vi "Sub Super Duper_14_02_12_JWa.vi"(0 "VISA resource name":refnum<visa-resource-name>="GPIB0::17::INSTR", 1 "Sample Properties:":T9 {"Date Created" format="%<%Y/%m/%d>T"}, 2 "Gated SMU4 is...":bool, 3 "TRF Cluster":T10={"Step 4"=-38.0, "# of Loops"=1.0, "Transfer 2"=FALSE, "Start 4"=-2.0, "Total Points 2"=2, "Start 3"=40.0, "Stop 2"=-40.0, "Step 3"=-1.0, "Loop Step"=0.0, "Integration Time 3"=0, "Loop Wait"=0.0, "First Step"=0.0} {"Loop Wait" format="%<%H:%M:%S>t"; "Integration Time 3" scale=0.0..2.0; "Step 3" format="%.2f"; "Stop 2" format="%.2f"; "Start 3" format="%.2f"; "Start 4" format="%.2f"; "Step 4" format="%.2f"}, 4 "TSP Cluster":T11={"Transport"=FALSE, "Start 2"=0.0, "Stop 3"=-60.0, "Step 2"=-1.0, "Start"=0.0, "Step"=-10.0, "Total Points"=7, "Integration Time"=0} {"Integration Time" scale=0.0..2.0; "Step" format="%.2f"; "Start" format="%.2f"; "Step 2" format="%.2f"; "Stop 3" format="%.2f"; "Start 2" format="%.2f"}, 5 "Compliance Cluster":T6={"Var1 sweep settings"={"sweep spacing (linear: 0)"=0, "sweep mode"=FALSE, "compliance (V)"=100.0, "compliance (A)"=0.001}, "Var1 sweep settings 2"={"sweep spacing (linear: 0)"=0, "sweep mode"=FALSE, "compliance (V)"=100.0, "compliance (A)"=0.001}, "Var2 step settings 2"={"compliance (A)"=0.001, "compliance (V)"=100.0}, "Var2 step settings"={"compliance (A)"=0.001, "compliance (V)"=100.0}} {"Var2 step settings"."compliance (V)" format="%.2f"; "Var2 step settings"."compliance (A)" format="%^.2e"; "Var2 step settings 2"."compliance (V)" format="%.2f"; "Var2 step settings 2"."compliance (A)" format="%^.2e"; "Var1 sweep settings 2"."compliance (A)" format="%^.2e"; "Var1 sweep settings 2"."compliance (V)" format="%.2f"; "Var1 sweep settings 2"."sweep spacing (linear: 0)" items=["linear", "log 10", "log 25", "log 50"]; "Var1 sweep settings"."compliance (A)" format="%^.2e"; "Var1 sweep settings"."compliance (V)" format="%.2f"; "Var1 sweep settings"."sweep spacing (linear: 0)" items=["linear", "log 10", "log 25", "log 50"]}, 6 "Light Bathe Cluster":T2={"TG to BG:  "=FALSE, "TG to BG Durration"=120.0, "TRF to TSP:   "=FALSE, "TRF to TSP Duration"=120.0, "Post Measure: "=FALSE, "TG to BG (TSP):"=FALSE, "TG to BG Durration 3"=120.0} {"TG to BG Durration 3" format="%<%H:%M:%S>t"; "TRF to TSP Duration" format="%<%H:%M:%S>t"; "TG to BG Durration" format="%<%H:%M:%S>t"}, 7 "error in":errorcluster, 8 "Saved Folder:":path=path "C:/1DATA/2011", 9 "Wait Cluster":T5 {"Wait Time (s)" format="%.1g"; "Wait Countdown" format="%<%H:%M:%S%1u>t"}, 13 "Stop \nCountdown":bool, 15 "Loop Count":dbl, 16 "Gate Current Cluster":T3={"Gate Current (TSP)"={"Y2 axis on/off"=FALSE, "MINIMUM"=0.0, "MAXIMUM"=1.0, "Variable name"="Ig", "LIN or LOG axis"="LIN"}, "Gate Current (TRF)"={"Y2 axis on/off"=FALSE, "MINIMUM"=0.0, "MAXIMUM"=1.0, "Variable name"="Ig", "LIN or LOG axis"="LIN"}} {"Gate Current (TSP)"."MAXIMUM" format="%.9f"; "Gate Current (TSP)"."MINIMUM" format="%.9f"; "Gate Current (TRF)"."MAXIMUM" format="%.9f"; "Gate Current (TRF)"."MINIMUM" format="%.9f"}, 17 "Dielectric Constant (BG)":dbl) -> (12 "Status Indicator":bool, 14 "Vt Cluster":T4 {"Id Max" format="%.3g"; "Vt Max" format="%.3g"; "Vt Min" format="%.3g"; "Vt Ratio" format="%.3g"}, 20 "VISA resource name out":refnum<visa-resource-name>, 21 "TRF Path":path, 23 "TSP Path":path, 24 "Graph Cluster":T7, 25 "Char Cluster":T8 {"Mobility-Lin" format="%#_4e"; "On/Off" format="%#_4e"; "Mobility-Sat" format="%#_4e"}, 27 "error out":errorcluster)   [LabVIEW 2012]
uses:
  <vilib>/Platform/TimedLoop/XDataNode/wakeup.ctl
  <vilib>/Platform/TimedLoop/XDataNode/XDNodeRunTimeDep.lvlib
  <vilib>/Platform/TimedLoop/XDataNode/nitl_modes.ctl
  <vilib>/Platform/TimedLoop/XDataNode/timing_clust.ctl
  <vilib>/Platform/TimedLoop/XDataNode/XDataNode.xnode
panel:
  in  "TG Dielectric Prop":T1
  out "LKG Path":path
  # "Vg Sweep"
  # "Vd Step"
  # "Loops and Integration Time"
  # "Device Characteristics"
  # "Light Bath is..."
  # "Duration (hh:mm:ss)"
  # "Sample Properties:"
  # "%"
  # "nm"
  # "Device Properties:"
  # "um"
  # "um"
  # "Vg Step"
  # "Vd Step"
  # "Integration Time"
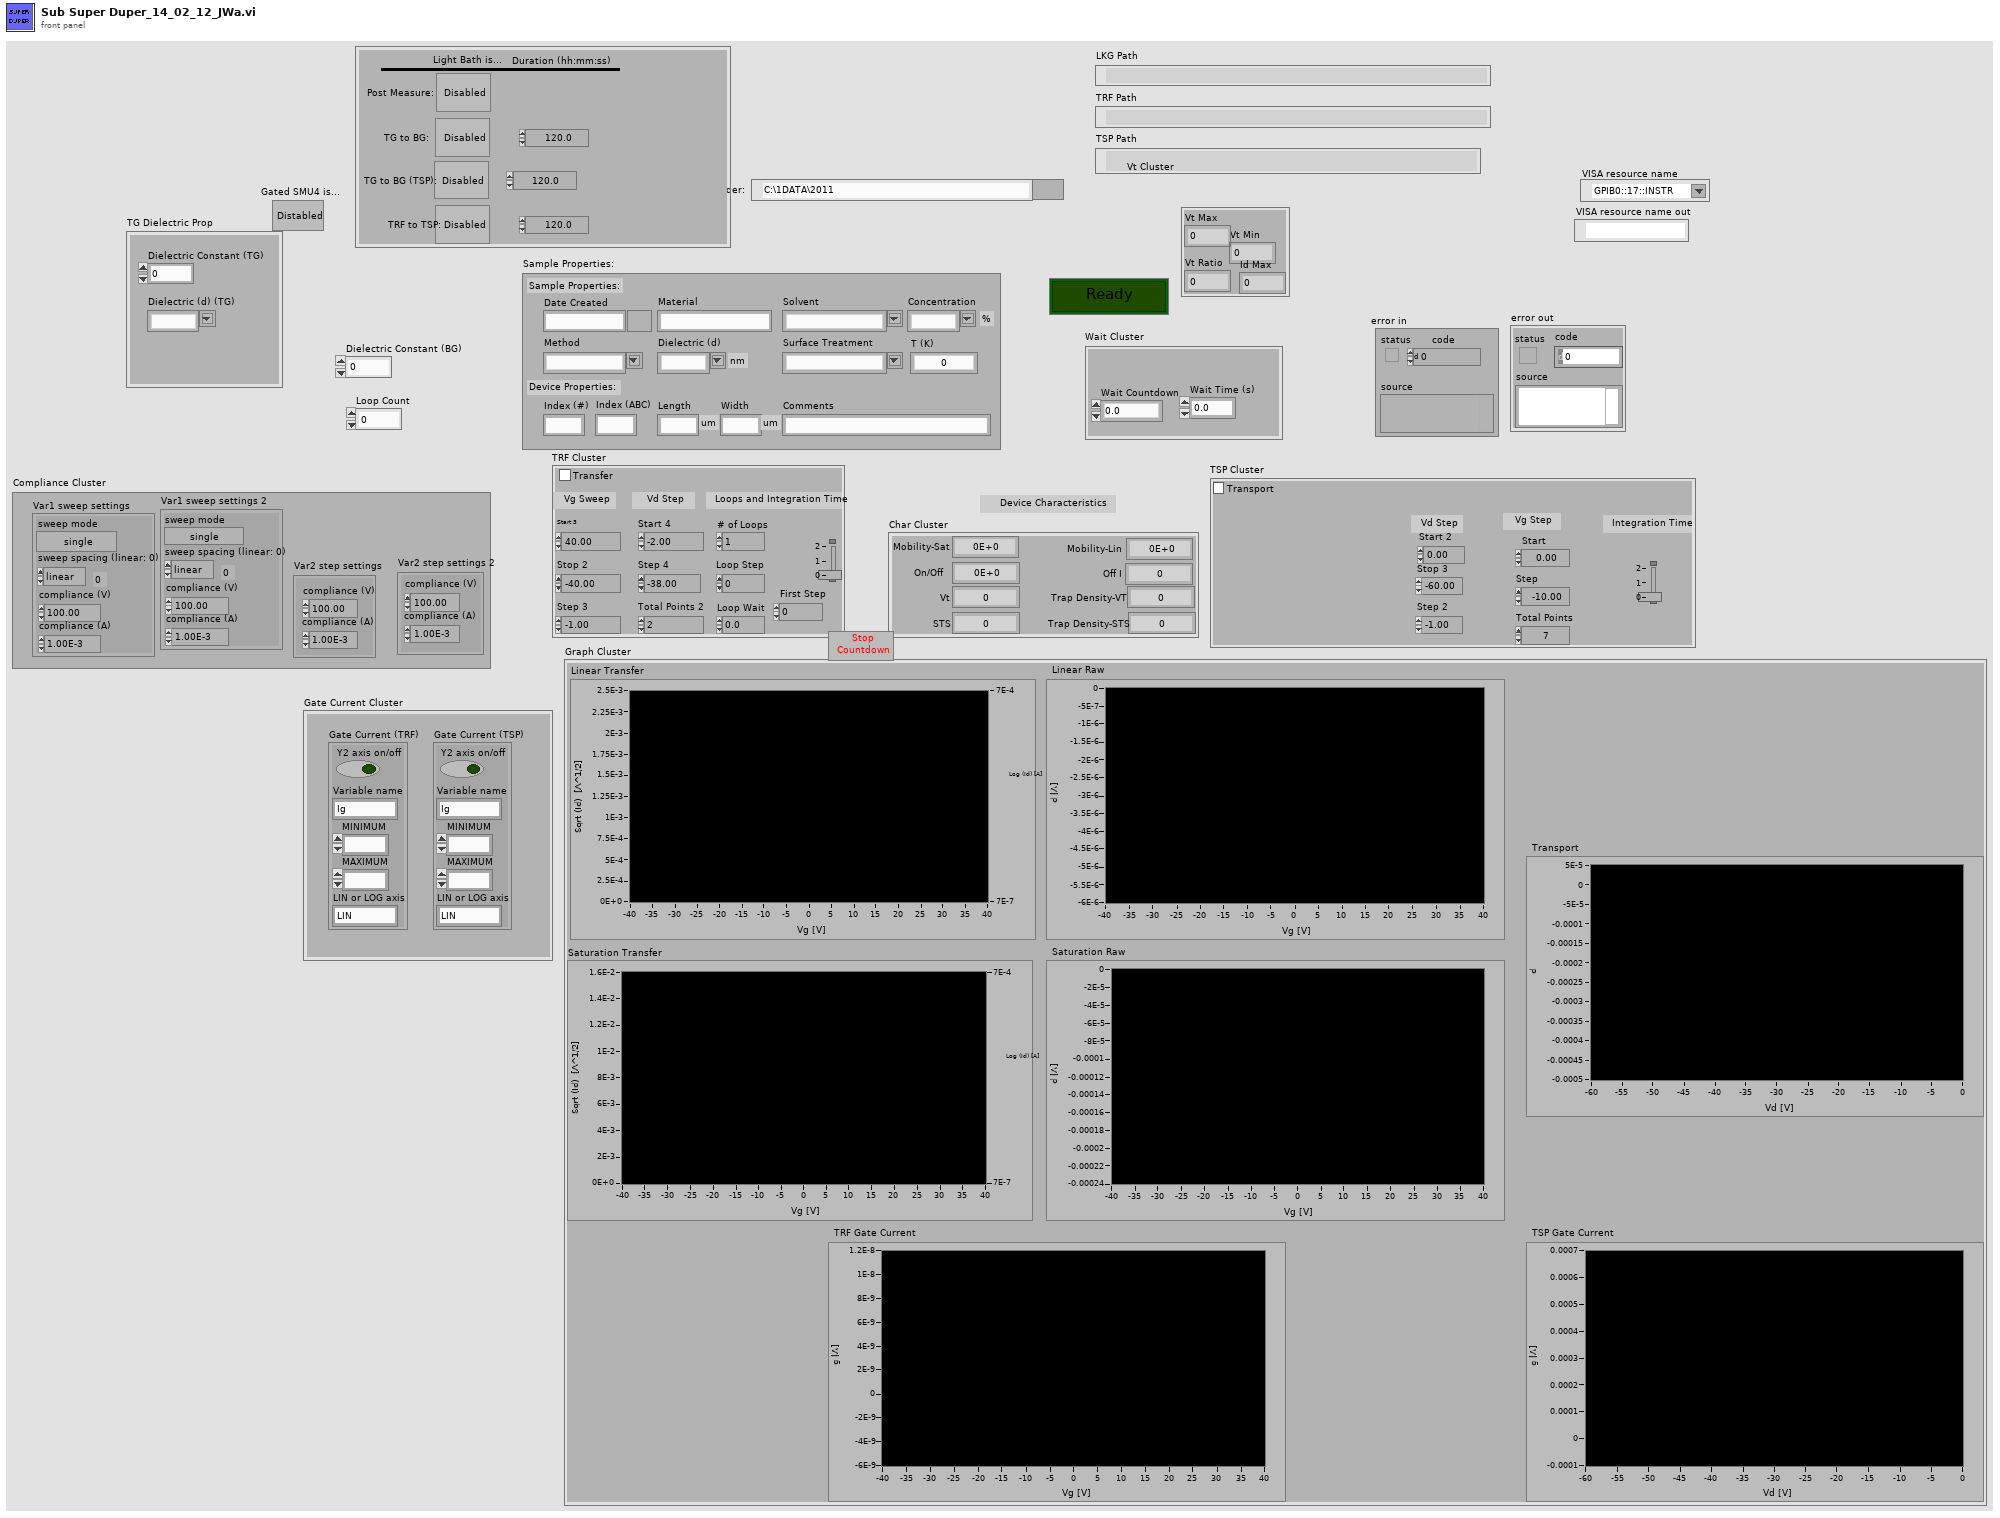
[diagram p1: front panel]
types:
  T1 = cluster{"Dielectric Constant (TG)":dbl, "Dielectric (d) (TG)":string}
  T2 = cluster{"TG to BG:  ":bool, "TG to BG Durration":dbl, "TRF to TSP:   ":bool, "TRF to TSP Duration":dbl, "Post Measure: ":bool, "TG to BG (TSP):":bool, "TG to BG Durration 3":dbl}
  T3 = cluster{"Gate Current (TSP)":cluster{"Y2 axis on/off":bool, "MINIMUM":ext, "MAXIMUM":ext, "Variable name":string, "LIN or LOG axis":string}, "Gate Current (TRF)":cluster{"Y2 axis on/off":bool, "MINIMUM":ext, "MAXIMUM":ext, "Variable name":string, "LIN or LOG axis":string}}
  T4 = cluster{"Vt Max":i32, "Vt Min":i32, "Vt Ratio":i32, "Id Max":i32}
  T5 = cluster{"Wait Countdown":dbl, "Wait Time (s)":dbl}
  T6 = cluster{"Var1 sweep settings":cluster{"sweep spacing (linear: 0)":u16, "sweep mode":bool, "compliance (V)":dbl, "compliance (A)":dbl}, "Var1 sweep settings 2":cluster{"sweep spacing (linear: 0)":u16, "sweep mode":bool, "compliance (V)":dbl, "compliance (A)":dbl}, "Var2 step settings 2":cluster{"compliance (A)":dbl, "compliance (V)":dbl}, "Var2 step settings":cluster{"compliance (A)":dbl, "compliance (V)":dbl}}
  T7 = cluster{"Linear Transfer":cluster{dbl[], "trace":dbl[]}[], "Linear Raw":cluster{dbl[], dbl[]}[], "Saturation Transfer":cluster{dbl[], "trace":dbl[]}[], "Saturation Raw":cluster{dbl[], dbl[]}[], "Transport":cluster{dbl[], dbl[]}[], "TRF Gate Current":cluster{dbl[], dbl[]}[], "TSP Gate Current":cluster{dbl[], dbl[]}[]}
  T8 = cluster{"Mobility-Sat":dbl, "Mobility-Lin":dbl, "On/Off ":dbl, "Off I":dbl, "Vt":dbl, "STS":dbl, "Trap Density-VT":dbl, "Trap Density-STS":dbl}
  T9 = cluster{"Date Created":timestamp, "Material":string, "Solvent":string, "Concentration":string, "Method":string, "Dielectric (d)":string, "Index (#)":string, "Index (ABC)":string, "Length":string, "Width":string, "Surface Treatment":string, "Comments":string, "T (K)":dbl}
  T10 = cluster{"Step 4":dbl, "# of Loops":dbl, "Transfer 2":bool, "Start 4":dbl, "Total Points 2":u16, "Start 3":dbl, "Stop 2":dbl, "Step 3":dbl, "Loop Step":dbl, "Integration Time 3":u32, "Loop Wait":dbl, "First Step":dbl}
  T11 = cluster{"Transport":bool, "Start 2":dbl, "Stop 3":dbl, "Step 2":dbl, "Start":dbl, "Step":dbl, "Total Points":u16, "Integration Time":u32}
  T12 = typedef "XDNodeRunTimeDep.lvlib/timing_clust.ctl" = cluster{"Expected End [f-1]":u64, "Actual End [f-1]":u64, "Finished Late? [f-1]":bool, "Expected End [i-1]":u64, "Actual End [i-1]":u64, "Finished Late? [i-1]":bool, "Expected Start [i]":u64, "Actual Start [i]":u64, "Expected Start [f]":u64, "Actual Start [f]":u64, "Source Name":string, "Structure Name":string, "Period":i64, "Deadline":i64, "Offset":i64, "Start":i64, "Priority":i32, "Timeout":i32, "Mode":T13, "Wakeup Reason":T14, "Error":errorcluster, "Source Type":string, "Secondary Source Type":string, "Global End Time":u64, "Global Start Time":u64, "Frame Duration":u64, "Iteration Duration":u64, "Assigned CPU":i32, "I/O Scan Engine Mode":u32}
  T13 = typedef "XDNodeRunTimeDep.lvlib/nitl_modes.ctl" = enum32{"No Change", "Process missed periods, maintain original phase", "Discard missed periods, maintain original phase", "Process missed periods, ignore original phase", "Discard missed periods, ignore original phase"}
  T14 = typedef "XDNodeRunTimeDep.lvlib/wakeup.ctl" = enum32{"Normal", "Aborted", "Asynchronous wakeup", "Timing source error", "Timed loop error", "Timeout"}
  T15 = cluster{"sweep spacing (linear: 0)":u16, "sweep mode":bool, "compliance (V)":dbl, "compliance (A)":dbl}
  T16 = cluster{"compliance (A)":dbl, "compliance (V)":dbl}
  T17 = cluster{"Y2 axis on/off":bool, "MINIMUM":ext, "MAXIMUM":ext, "Variable name":string, "LIN or LOG axis":string}
  T18 = cluster{"Start 3":dbl, "Stop 2":dbl, "Step 3":dbl, "sweep spacing (linear: 0)":u16, "sweep mode":bool, "compliance (V)":dbl, "compliance (A)":dbl}
  T19 = cluster{"compliance (A)":dbl, "compliance (V)":dbl, "Start 4":dbl, "Total Points 2":u16, dbl}
  T20 = cluster{"Vt Max":i32, "Vt Min":i32, "Vt Ratio":i32, "Id Max":dbl}
  T21 = cluster{"Mobility-Sat":dbl, "Mobility-Lin":dbl, "On/Off Current":dbl, "Off I":dbl, "Vt":dbl, "STS":dbl, "Trap Density-VT":dbl, "Trap Density-STS":dbl}
  T22 = cluster{"Linear Sqrt":cluster{dbl[], "trace":dbl[]}[], "Linear Log":cluster{dbl[], "trace":dbl[]}[], "Linear Raw":cluster{dbl[], dbl[]}[], "Saturation Sqrt":cluster{dbl[], "trace":dbl[]}[], "Saturation Log":cluster{dbl[], "trace":dbl[]}[], "Saturation Raw":cluster{dbl[], "trace":dbl[]}[], "Gate Current":cluster{dbl[], "trace":dbl[]}[]}
  T23 = cluster{"Start 2":dbl, "Stop 3":dbl, "Step 2":dbl, "sweep spacing (linear: 0)":u16, "sweep mode":bool, "compliance (V)":dbl, "compliance (A)":dbl}
  T24 = cluster{"compliance (A)":dbl, "compliance (V)":dbl, "Start":dbl, "Total Points":u16, "Step":dbl}
  T25 = cluster{"Transport":cluster{dbl[], dbl[]}[], "Gate Current":cluster{dbl[], dbl[]}[]}
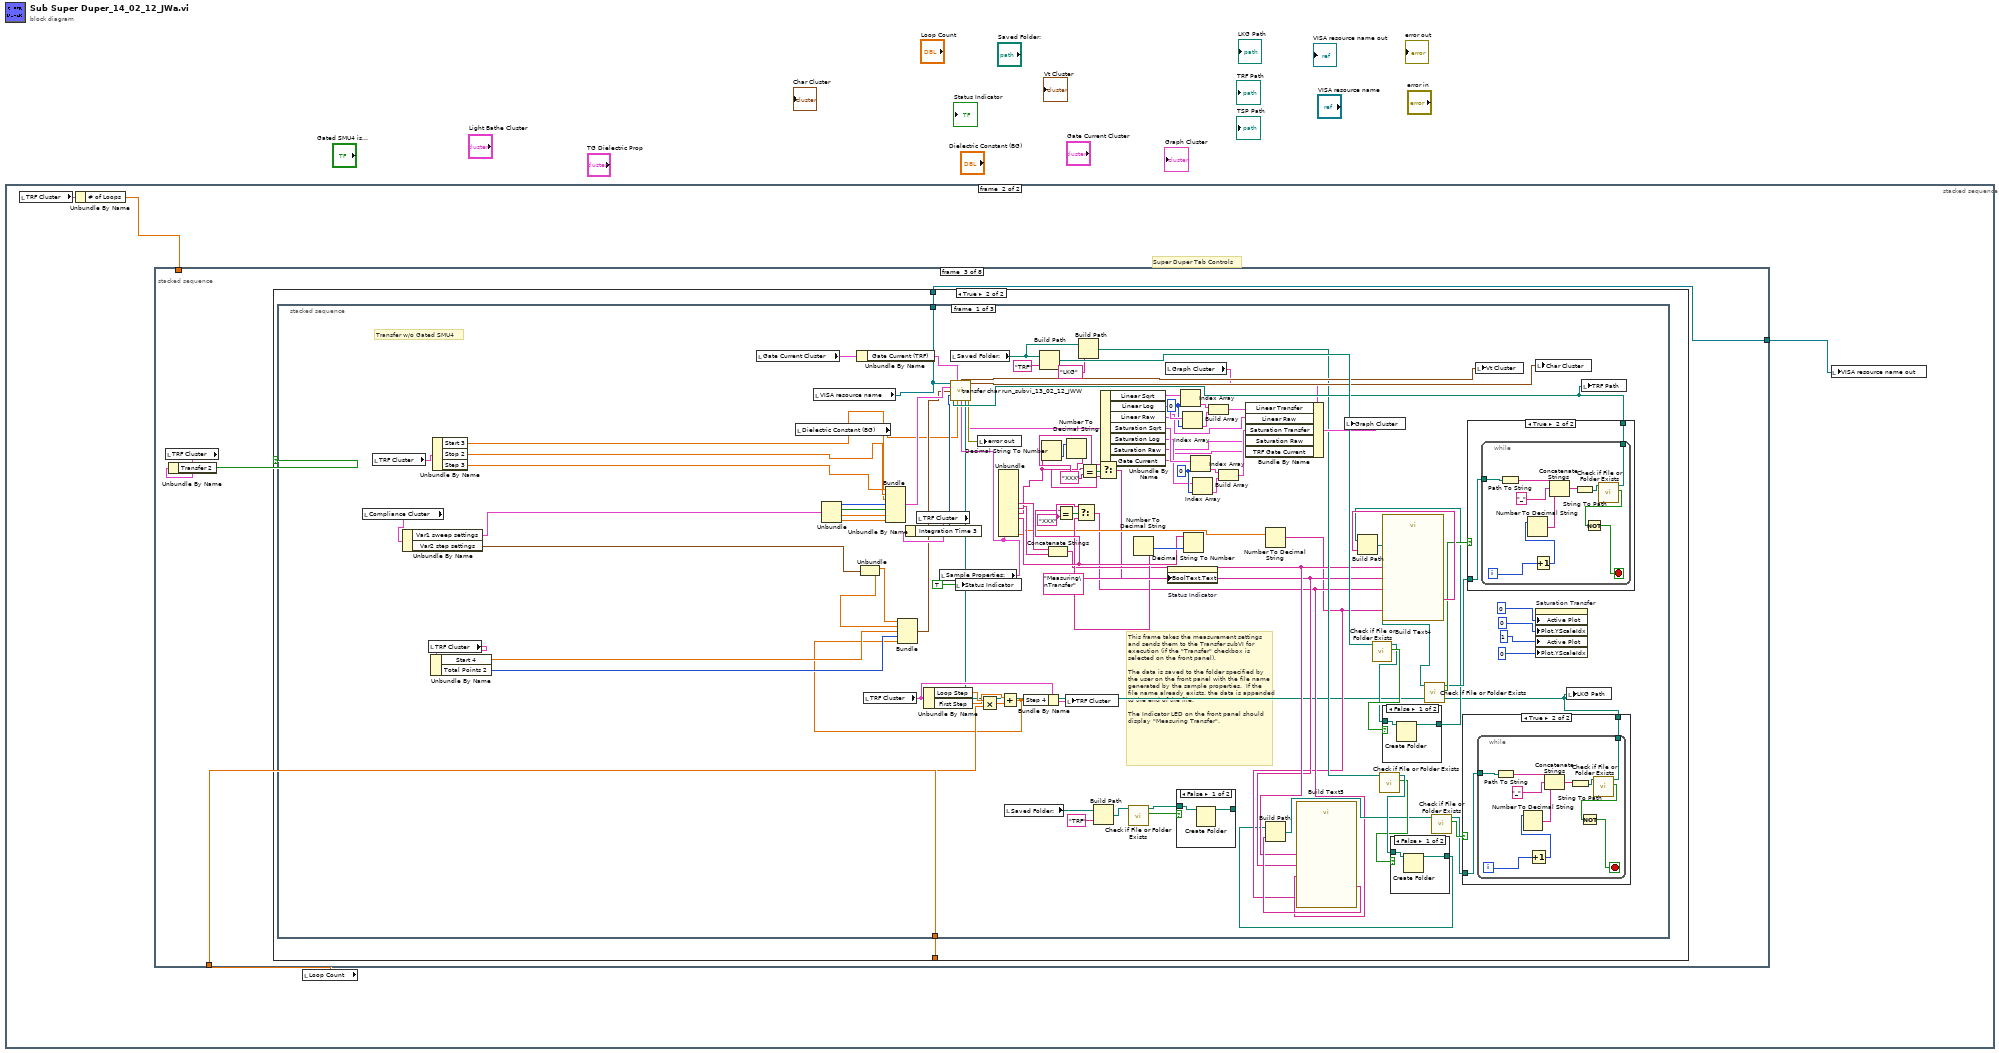
[diagram p0: block diagram]
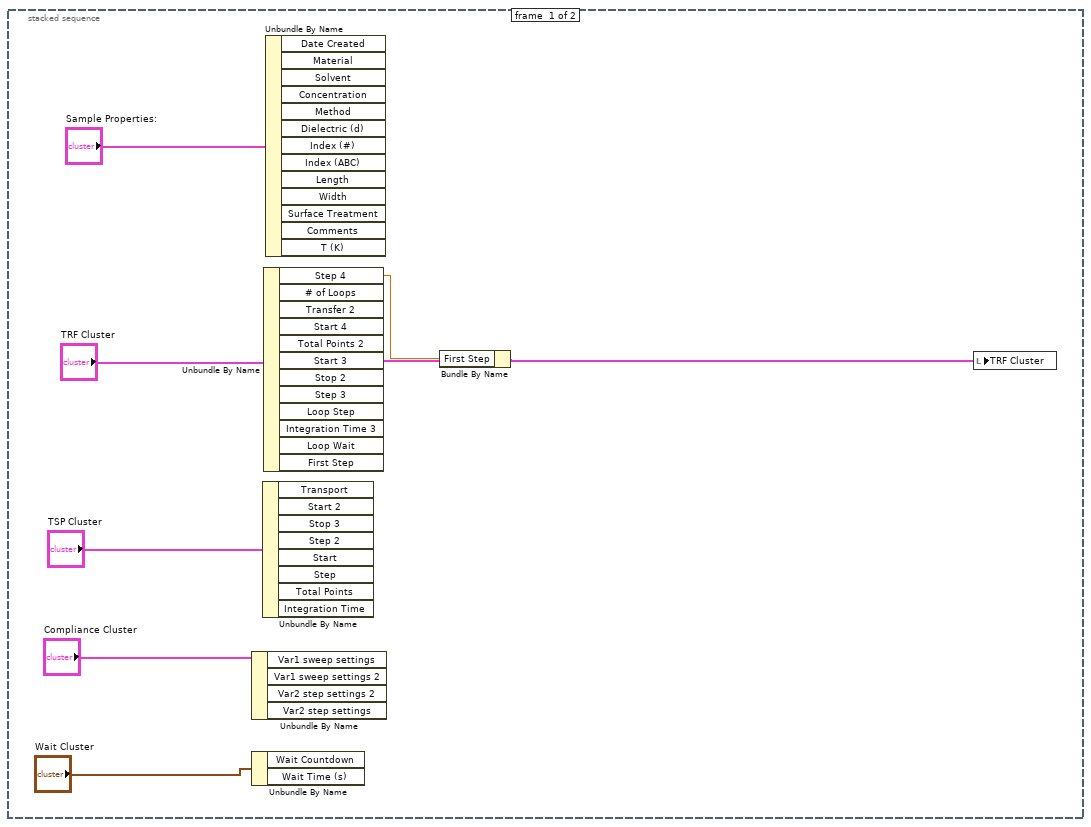
[diagram p2: hidden frame]
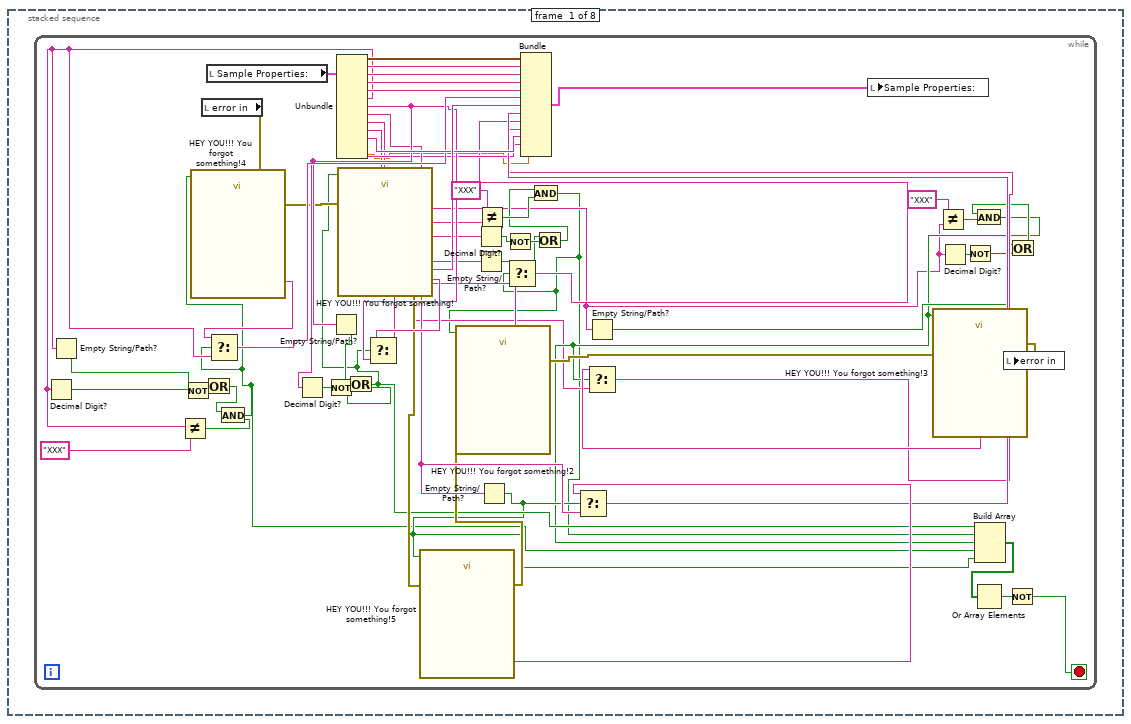
[diagram p3: hidden frame]
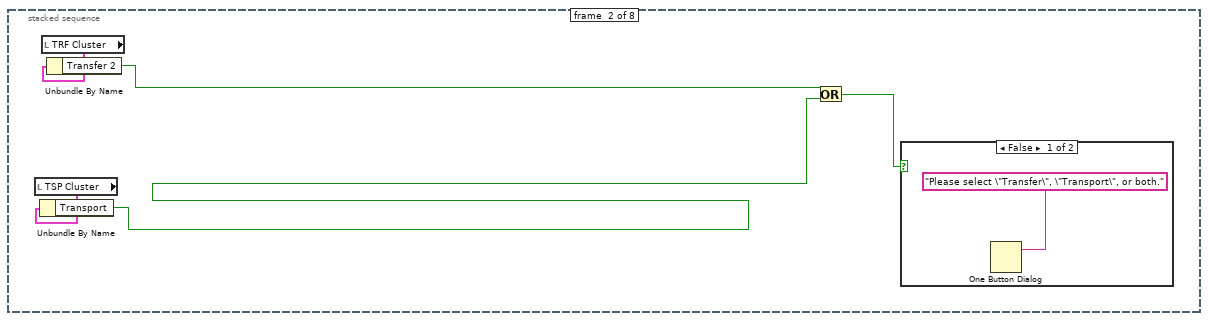
[diagram p4: hidden frame]
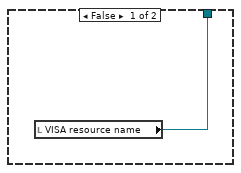
[diagram p6: hidden frame]
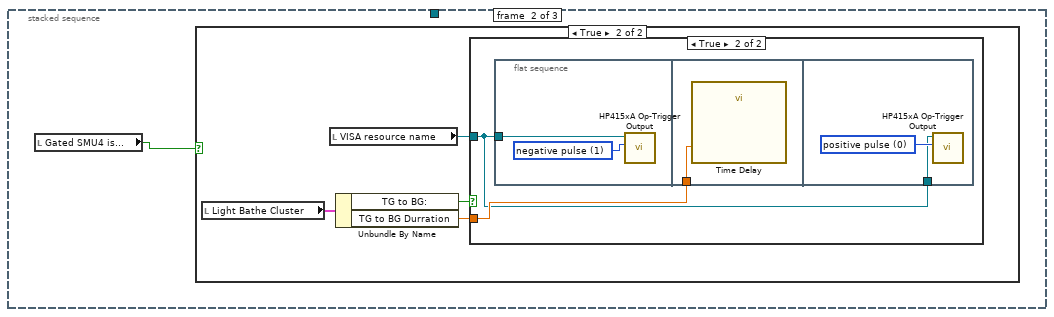
[diagram p12: hidden frame]
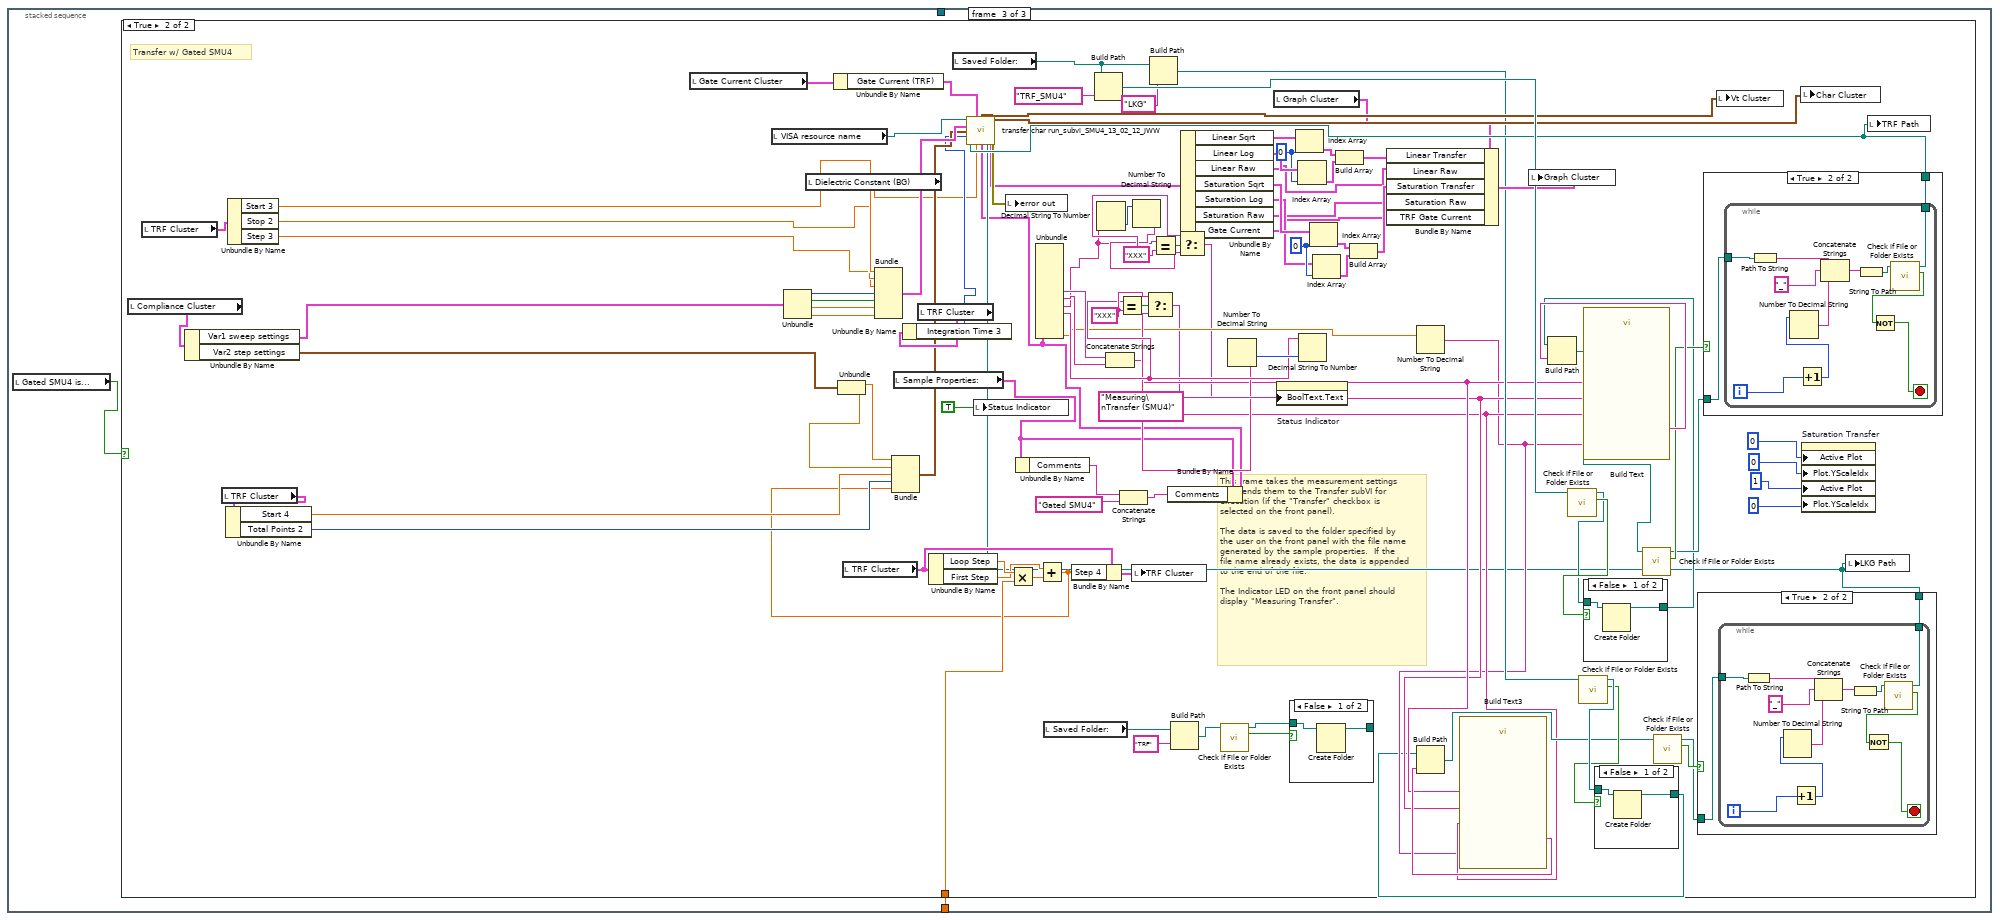
[diagram p15: hidden frame]
diagram:
  n1 = stacked-sequence {
    frame #0 {
      n2 = Unbundle By Name("Compliance Cluster") -> ()  [unwired: 4 out]
      n3 = Unbundle By Name("Wait Cluster") -> ()  [unwired: 2 out]
      n4 = Unbundle By Name("TSP Cluster") -> ()  [unwired: 8 out]
      n5 = Unbundle By Name("TRF Cluster") -> ("Step 4"=w7:dbl)  [unwired: 11 out]
      n6 = Unbundle By Name("Sample Properties:") -> ()  [unwired: 13 out]
      n7 = Bundle By Name(cluster="TRF Cluster", "First Step"=w7) -> (w5:T10)
      n8 = local write "TRF Cluster"(w5) -> ()
    }
    frame #1 {
      # "Super Duper Tab Controls"
      n9 = local read "TRF Cluster"() -> (w11:T10)
      n10 = Unbundle By Name(w11) -> ("# of Loops"=w10:dbl)
      n11 = local read "Loop Count"() -> (w8:dbl)
      n12 = stacked-sequence {
        tunnel: w8 -> [_ _ w81 _ _ _ _ w593]
        tunnel: w10 -> [_ _ _ _ _ _ _ w592]
        tunnel: [_ _ w78 _ _ _ _ _] -> w9
        frame #0 {
          n13 = while {
            stop <- w37 stop-if-true
            n14 = local read "error in"() -> (w43:errorcluster)
            n15 = local read "Sample Properties:"() -> (w66:T9)
            n16 = Unbundle(w66) -> ("Date Created"=w67:timestamp, "Material"=w68:string, "Solvent"=w69:string, "Concentration"=w70:string, "Method"=w71:string, "Dielectric (d)"=w26:string, "Index (#)"=w56:string, "Index (ABC)"=w53:string, "Length"=w21:string, "Width"=w14:string, "Surface Treatment"=w59:string, "Comments"=w51:string, "T (K)"=w12:dbl)
            n17 = Decimal Digit?(1:w26) -> (0:w34:bool)
            n18 = Empty String/Path?(string/path=w26) -> (empty?=w28:bool)
            n19 = Not Equal?(x=w26, y="XXX") -> (x != y?=w25:bool)
            n20 = Not(x=w34) -> (.not. x?=w31:bool)
            n21 = Or(x=w28, y=w31) -> (x .or. y?=w24:bool)
            n22 = And(x=w24, y=w25) -> (x .and. y?=w23:bool)
            n23 = call "HEY YOU!!! You forgot something!4"("Enable"=w23, "error in (no error)"=w43) -> ("Dielectric (d)"=w58:string, "error out"=w42:errorcluster)  [unwired: 15 in, 1 out]
            n24 = Select(t=w58, s=w23, f=w26) -> (s? t:f=w57:string)
            n25 = Decimal Digit?(1:w56) -> (0:w47:bool)
            n26 = Not(x=w47) -> (.not. x?=w46:bool)
            n27 = Empty String/Path?(string/path=w56) -> (empty?=w55:bool)
            n28 = Or(x=w55, y=w46) -> (x .or. y?=w41:bool)
            n29 = call "HEY YOU!!! You forgot something!"("Enable"=w41, "error in (no error)"=w42) -> ("Index (#)"=w65:string, "error out"=w45:errorcluster)  [unwired: 15 in, 1 out]
            n30 = Select(t=w65, s=w41, f=w56) -> (s? t:f=w62:string)
            n31 = Decimal Digit?(1:w21) -> (0:w36:bool)
            n32 = Empty String/Path?(string/path=w21) -> (empty?=w30:bool)
            n33 = Not Equal?(x="XXX", y=w21) -> (x != y?=w20:bool)
            n34 = Empty String/Path?(string/path=w53) -> (empty?=w40:bool)
            n35 = call "HEY YOU!!! You forgot something!5"("Enable"=w40, "error in (no error)"=w45) -> ("Index (ABC)"=w54:string, "error out"=w44:errorcluster)  [unwired: 15 in, 1 out]
            n36 = Not(x=w36) -> (.not. x?=w33:bool)
            n37 = Or(x=w30, y=w33) -> (x .or. y?=w19:bool)
            n38 = And(x=w19, y=w20) -> (x .and. y?=w13:bool)
            n39 = call "HEY YOU!!! You forgot something!2"("Enable"=w13, "error in (no error)"=w44) -> ("Length"=w64:string, "error out"=w61:errorcluster)  [unwired: 15 in, 1 out]
            n40 = Select(t=w64, s=w13, f=w21) -> (s? t:f=w50:string)
            n41 = Select(t=w54, s=w40, f=w53) -> (s? t:f=w52:string)
            n42 = Empty String/Path?(string/path=w14) -> (empty?=w29:bool)
            n43 = Not Equal?(x="XXX", y=w14) -> (x != y?=w18:bool)
            n44 = Decimal Digit?(1:w14) -> (0:w35:bool)
            n45 = Not(x=w35) -> (.not. x?=w32:bool)
            n46 = Or(x=w29, y=w32) -> (x .or. y?=w17:bool)
            n47 = And(x=w17, y=w18) -> (x .and. y?=w16:bool)
            n48 = call "HEY YOU!!! You forgot something!3"("Enable"=w16, "error in (no error)"=w61) -> ("Width"=w63:string, "error out"=w60:errorcluster)  [unwired: 15 in, 1 out]
            n49 = Select(t=w63, s=w16, f=w14) -> (s? t:f=w49:string)
            n50 = Bundle("Date Created"=w67, "Material"=w68, "Solvent"=w69, "Concentration"=w70, "Method"=w71, "Dielectric (d)"=w57, "Index (#)"=w62, "Index (ABC)"=w52, "Length"=w50, "Width"=w49, "Surface Treatment"=w59, "Comments"=w51, "T (K)"=w12) -> (w48:T9)  [unwired: 1 in]
            n51 = local write "Sample Properties:"(w48) -> ()
            n52 = Build Array(w41, w13, w16, w23, w40) -> (w39:bool[])
            n53 = Or Array Elements(Boolean array=w39) -> (logical OR=w38:bool)
            n54 = local write "error in"(w60) -> ()
            n55 = Not(x=w38) -> (.not. x?=w37:bool)
          }
        }
        frame #1 {
          n56 = local read "TSP Cluster"() -> (w73:T11)
          n57 = Unbundle By Name(w73) -> ("Transport"=w72:bool)
          n58 = local read "TRF Cluster"() -> (w75:T10)
          n59 = Unbundle By Name(w75) -> ("Transfer 2"=w74:bool)
          n60 = Or(x=w74, y=w72) -> (x .or. y?=w76:bool)
          n61 = case shown="False" w76 {
            frame False {
              n62 = One Button Dialog(message="Please select \"Transfer\", \"Transport\", or both.") -> ()  [unwired: 1 in, 1 out]
            }
            frame True {
            }
          }
        }
        frame #2 {
          n63 = local read "TRF Cluster"() -> (w79:T10)
          n64 = Unbundle By Name(w79) -> ("Transfer 2"=w80:bool)
          n65 = case shown="True" w80 {
            tunnel: w81 -> [_ w84]
            tunnel: [w82 w83] -> w78
            frame False {
              n66 = local read "VISA resource name"() -> (w82:refnum<visa-resource-name>)
            }
            frame True {
              n67 = stacked-sequence {
                tunnel: w84 -> [w186 _ w237]
                tunnel: [w185 _ _] -> w83
                frame #0 {
                  w115 = 0
                  w121 = 0
                  w164 = "XXX"
                  w167 = "XXX"
                  # "Transfer w/o Gated SMU4"
                  # "This frame takes the measurement settings and sends them to the Transfer subVI for execution (if the \"Transfer\" checkbox is selected on the front panel).\n\nThe data is saved to the folder specified by the user on the front panel with the file name generated by the sample properties.  If the file name already exists, the data is appended to the end of the file.\n\nThe Indicator LED on the front panel should display \"Measuring Transfer\"."
                  n68 = local read "Compliance Cluster"() -> (w143:T6)
                  n69 = local read "TRF Cluster"() -> (w148:T10)
                  n70 = Unbundle By Name(w143) -> ("Var1 sweep settings"=w141:T15, "Var2 step settings"=w142:T16)
                  n71 = local read "TRF Cluster"() -> (w151:T10)
                  n72 = Unbundle By Name(w151) -> ("Start 4"=w150:dbl, "Total Points 2"=w149:u16)
                  n73 = Unbundle By Name(w148) -> ("Start 3"=w147:dbl, "Stop 2"=w146:dbl, "Step 3"=w145:dbl)
                  n74 = local read "Gate Current Cluster"() -> (w87:T3)
                  n75 = local read "Dielectric Constant (BG)"() -> (w85:dbl)
                  n76 = local read "VISA resource name"() -> (w185:refnum<visa-resource-name>)
                  n77 = Unbundle(w141) -> ("sweep spacing (linear: 0)"=w184:u16, "sweep mode"=w183:bool, "compliance (V)"=w182:dbl, "compliance (A)"=w181:dbl)
                  n78 = Unbundle By Name(w87) -> ("Gate Current (TRF)"=w86:T17)
                  n79 = Unbundle(w142) -> ("compliance (A)"=w180:dbl, "compliance (V)"=w179:dbl)
                  n80 = local read "TRF Cluster"() -> (w134:T10)
                  n81 = Bundle("Start 3"=w147, "Stop 2"=w146, "Step 3"=w145, "sweep spacing (linear: 0)"=w184, "sweep mode"=w183, "compliance (V)"=w182, "compliance (A)"=w181) -> (w133:T18)  [unwired: 1 in]
                  n82 = local read "TRF Cluster"() -> (w144:T10)
                  n83 = Unbundle By Name(w144) -> ("Integration Time 3"=w131:u32)
                  n84 = Unbundle By Name(w134) -> ("Loop Step"=w137:dbl, "First Step"=w136:dbl)
                  n85 = local read "Sample Properties:"() -> (w129:T9)
                  n86 = local read "Saved Folder:"() -> (w102:path)
                  n87 = local write "Status Indicator"(TRUE) -> ()
                  n88 = Multiply(x=w137, y=w186) -> (x*y=w139:dbl)
                  n89 = Unbundle(w129) -> ("Index (#)"=w175:string, "Index (ABC)"=w174:string, "Length"=w161:string, "Width"=w163:string, "T (K)"=w140:dbl)  [unwired: 8 out]
                  n90 = Add(x=w136, y=w139) -> (x+y=w135:dbl)
                  n91 = Bundle("compliance (A)"=w180, "compliance (V)"=w179, "Start 4"=w150, "Total Points 2"=w149, w135) -> (w132:T19)  [unwired: 1 in]
                  n92 = local read "Saved Folder:"() -> (w108:path)
                  n93 = Bundle By Name(cluster=w134, "Step 4"=w135) -> (w138:T10)
                  n94 = Build Path(base path=w102, name or relative path="TRF") -> (appended path=w157:path)
                  n95 = Decimal String To Number(string=w161) -> (number=w170:i32)  [unwired: 2 in, 1 out]
                  n96 = Concatenate Strings(w175, w174) -> (w93:string)
                  n97 = Equal?(x=w163, y=w164) -> (x = y?=w165:bool)
                  n98 = local write "TRF Cluster"(w138) -> ()
                  n99 = Number To Decimal String(number=w170) -> (decimal integer string=w166:string)  [unwired: 1 in]
                  n100 = Build Path(base path=w102, name or relative path="LKG") -> (appended path=w98:path)
                  n101 = Equal?(x=w161, y=w167) -> (x = y?=w168:bool)
                  n102 = Build Path(base path=w108, name or relative path="TRF") -> (appended path=w106:path)
                  n103 = Select(t=w167, s=w168, f=w166) -> (s? t:f=w92:string)
                  n104 = call <vilib>:"Check if File or Folder Exists.vi"("path"=w106) -> ("file or folder exists?"=w104:bool, "dup path"=w105:path)  [unwired: 8 in, 1 out]
                  n105 = local read "Graph Cluster"() -> (w124:T7)
                  n106 = property on="Status Indicator" class="Bool (strict)"("BoolText.Text"="Measuring\nTransfer") -> ()  [unwired: 2 in, 2 out]
                  n107 = case shown="False" w104 {
                    tunnel: w105 -> [w205 w206]
                    tunnel: [w204 w206] -> _
                    frame False {
                      n108 = Create Folder(path (use dialog)=w205) -> (created path=w204:path)  [unwired: 2 in, 2 out]
                    }
                    frame True {
                    }
                  }
                  n109 = Decimal String To Number(string=w163) -> (number=w169:i32)  [unwired: 2 in, 1 out]
                  n110 = Number To Decimal String(number=w169) -> (decimal integer string=w162:string)  [unwired: 1 in]
                  n111 = Select(t=w164, s=w165, f=w162) -> (s? t:f=w91:string)
                  n112 = Number To Decimal String(number=w140) -> (decimal integer string=w90:string)  [unwired: 1 in]
                  n113 = call "Build Text5"("T"=w90, "Index"=w93, "Length"=w92, "Width"=w91) -> ("Result"=w94:string)  [unwired: 10 in, 1 out]
                  n114 = call <vilib>:"Check if File or Folder Exists.vi"("path"=w157) -> ("file or folder exists?"=w159:bool, "dup path"=w158:path)  [unwired: 8 in, 1 out]
                  n115 = call <vilib>:"Check if File or Folder Exists.vi"("path"=w98) -> ("file or folder exists?"=w99:bool, "dup path"=w100:path)  [unwired: 8 in, 1 out]
                  n116 = call "Build Text4"("T"=w90, "Index"=w93, "Length"=w92, "Width"=w91) -> ("Result"=w178:string)  [unwired: 10 in, 1 out]
                  n117 = case shown="False" w159 {
                    tunnel: w158 -> [w208 w209]
                    tunnel: [w207 w209] -> w156
                    frame False {
                      n118 = Create Folder(path (use dialog)=w208) -> (created path=w207:path)  [unwired: 2 in, 2 out]
                    }
                    frame True {
                    }
                  }
                  n119 = Build Path(base path=w156, name or relative path=w178) -> (appended path=w172:path)
                  n120 = case shown="False" w99 {
                    tunnel: w100 -> [w202 w203]
                    tunnel: [w201 w203] -> w89
                    frame False {
                      n121 = Create Folder(path (use dialog)=w202) -> (created path=w201:path)  [unwired: 2 in, 2 out]
                    }
                    frame True {
                    }
                  }
                  n122 = Build Path(base path=w89, name or relative path=w94) -> (appended path=w97:path)
                  n123 = call <vilib>:"Check if File or Folder Exists.vi"("path"=w172) -> ("file or folder exists?"=w173:bool, "dup path"=w171:path)  [unwired: 8 in, 1 out]
                  n124 = call <vilib>:"Check if File or Folder Exists.vi"("path"=w97) -> ("file or folder exists?"=w96:bool, "dup path"=w95:path)  [unwired: 8 in, 1 out]
                  n125 = case shown="True" w96 {
                    tunnel: w95 -> [w187 w189]
                    tunnel: [w187 w188] -> w88
                    frame False {
                    }
                    frame True {
                      n126 = while {
                        tunnel: w189 -> [w191]
                        tunnel: [w190] -> w188
                        i -> [w193]
                        stop <- w194 stop-if-true
                        n127 = Path To String(path=w191) -> (string=w200:string)
                        n128 = Increment(x=w193) -> (x+1=w192:i32)
                        n129 = Number To Decimal String(number=w192) -> (decimal integer string=w198:string)  [unwired: 1 in]
                        n130 = Concatenate Strings(w200, "_", w198) -> (w197:string)
                        n131 = String To Path(string=w197) -> (path=w196:path)
                        n132 = call <vilib>:"Check if File or Folder Exists.vi"("path"=w196) -> ("file or folder exists?"=w195:bool, "dup path"=w190:path)  [unwired: 8 in, 1 out]
                        n133 = Not(x=w195) -> (.not. x?=w194:bool)
                      }
                    }
                  }
                  n134 = case shown="True" w173 {
                    tunnel: w171 -> [w210 w212]
                    tunnel: [w210 w211] -> w130
                    frame False {
                    }
                    frame True {
                      n135 = while {
                        tunnel: w212 -> [w214]
                        tunnel: [w213] -> w211
                        i -> [w216]
                        stop <- w217 stop-if-true
                        n136 = Path To String(path=w214) -> (string=w223:string)
                        n137 = Increment(x=w216) -> (x+1=w215:i32)
                        n138 = Number To Decimal String(number=w215) -> (decimal integer string=w221:string)  [unwired: 1 in]
                        n139 = Concatenate Strings(w223, "_", w221) -> (w220:string)
                        n140 = String To Path(string=w220) -> (path=w219:path)
                        n141 = call <vilib>:"Check if File or Folder Exists.vi"("path"=w219) -> ("file or folder exists?"=w218:bool, "dup path"=w213:path)  [unwired: 8 in, 1 out]
                        n142 = Not(x=w218) -> (.not. x?=w217:bool)
                      }
                    }
                  }
                  n143 = call "transfer char run_subvi_13_02_12_JWW.vi"("VISA session"=w185, "Y2 axis settings"=w86, "LKG Path"=w88, "Var1 sweep settings"=w133, "Var2 step settings"=w132, "integration time"=w131, "Input Path"=w130, "Dielectric Constant"=w85, "Sample Properties:"=w129) -> ("Check Cluster"=w126:T20, "Output"=w127:T21, "Graph Cluster"=w125:T22, "error?"=w128:errorcluster)  [unwired: 3 in]
                  n144 = local write "error out"(w128) -> ()
                  n145 = Unbundle By Name(w125) -> ("Linear Sqrt"=w123:cluster{dbl[], "trace":dbl[]}[], "Linear Log"=w122:cluster{dbl[], "trace":dbl[]}[], "Linear Raw"=w111:cluster{dbl[], dbl[]}[], "Saturation Sqrt"=w114:cluster{dbl[], "trace":dbl[]}[], "Saturation Log"=w113:cluster{dbl[], "trace":dbl[]}[], "Saturation Raw"=w110:cluster{dbl[], "trace":dbl[]}[], "Gate Current"=w103:cluster{dbl[], "trace":dbl[]}[])
                  n146 = Index Array(array=w123, index=w121) -> (element=w120:cluster{dbl[], "trace":dbl[]})
                  n147 = Index Array(array=w122, index=w121) -> (element=w119:cluster{dbl[], "trace":dbl[]})
                  n148 = Index Array(array=w114, index=w115) -> (element=w116:cluster{dbl[], "trace":dbl[]})
                  n149 = Index Array(array=w113, index=w115) -> (element=w117:cluster{dbl[], "trace":dbl[]})
                  n150 = Build Array(w120, w119) -> (w118:cluster{dbl[], "trace":dbl[]}[])
                  n151 = Build Array(w116, w117) -> (w112:cluster{dbl[], "trace":dbl[]}[])
                  n152 = Bundle By Name(cluster=w124, "Linear Transfer"=w118, "Linear Raw"=w111, "Saturation Transfer"=w112, "Saturation Raw"=w110, "TRF Gate Current"=w103) -> (w109:T7)
                  n153 = local write "Graph Cluster"(w109) -> ()
                  n154 = local write "Vt Cluster"(w126) -> ()
                  n155 = local write "Char Cluster"(w127) -> ()
                  n156 = property on="Saturation Transfer" class="XYGraph (strict)"("Active Plot"=0, "Plot.YScaleIdx"=0, "Active Plot"=1, "Plot.YScaleIdx"=0) -> ()  [unwired: 2 in, 2 out]
                  n157 = local write "LKG Path"(w88) -> ()
                  n158 = local write "TRF Path"(w130) -> ()
                }
                frame #1 {
                  n159 = local read "Gated SMU4 is..."() -> (w224:bool)
                  n160 = case shown="True" w224 {
                    frame False {
                    }
                    frame True {
                      n161 = local read "Light Bathe Cluster"() -> (w228:T2)
                      n162 = local read "VISA resource name"() -> (w225:refnum<visa-resource-name>)
                      n163 = Unbundle By Name(w228) -> ("TG to BG:"=w227:bool, "TG to BG Durration"=w226:dbl)
                      n164 = case shown="True" w227 {
                        tunnel: w226 -> [_ w230]
                        tunnel: w225 -> [_ w229]
                        frame False {
                        }
                        frame True {
                          n165 = flat-sequence {
                            tunnel: w229 -> [w231]
                            tunnel: w230 -> [w233]
                            tunnel: w229 -> [w234]
                            frame #0 {
                              w232 = u32 1 items=["positive pulse  ", "negative pulse  ", "level high  ", "level low  "] ("trigger signal")
                              n166 = call "HP415xA Op-Trigger Output.vi"("trigger signal"=w232, "VISA session"=w231) -> ()  [unwired: 2 in, 1 out]
                            }
                            frame #1 {
                              n167 = call "Time Delay"("Delay Time (s)"=w233) -> ()  [unwired: 10 in, 1 out]
                            }
                            frame #2 {
                              w235 = u32 0 items=["positive pulse  ", "negative pulse  ", "level high  ", "level low  "] ("trigger signal")
                              n168 = call "HP415xA Op-Trigger Output.vi"("trigger signal"=w235, "VISA session"=w234) -> ()  [unwired: 2 in, 1 out]
                            }
                          }
                        }
                      }
                    }
                  }
                }
                frame #2 {
                  n169 = local read "Gated SMU4 is..."() -> (w236:bool)
                  n170 = case shown="True" w236 {
                    tunnel: w237 -> [_ w297]
                    frame False {
                    }
                    frame True {
                      w273 = 0
                      w279 = 0
                      w323 = "XXX"
                      w326 = "XXX"
                      # "Transfer w/ Gated SMU4"
                      # "This frame takes the measurement settings and sends them to the Transfer subVI for execution (if the \"Transfer\" checkbox is selected on the front panel).\n\nThe data is saved to the folder specified by the user on the front panel with the file name generated by the sample properties.  If the file name already exists, the data is appended to the end of the file.\n\nThe Indicator LED on the front panel should display \"Measuring Transfer\"."
                      n171 = local read "Compliance Cluster"() -> (w302:T6)
                      n172 = local read "TRF Cluster"() -> (w307:T10)
                      n173 = Unbundle By Name(w302) -> ("Var1 sweep settings"=w300:T15, "Var2 step settings"=w301:T16)
                      n174 = local read "TRF Cluster"() -> (w310:T10)
                      n175 = Unbundle By Name(w310) -> ("Start 4"=w309:dbl, "Total Points 2"=w308:u16)
                      n176 = Unbundle By Name(w307) -> ("Start 3"=w306:dbl, "Stop 2"=w305:dbl, "Step 3"=w304:dbl)
                      n177 = local read "Gate Current Cluster"() -> (w245:T3)
                      n178 = local read "VISA resource name"() -> (w291:refnum<visa-resource-name>)
                      n179 = Unbundle(w300) -> ("sweep spacing (linear: 0)"=w343:u16, "sweep mode"=w342:bool, "compliance (V)"=w341:dbl, "compliance (A)"=w340:dbl)
                      n180 = local read "Dielectric Constant (BG)"() -> (w238:dbl)
                      n181 = Unbundle By Name(w245) -> ("Gate Current (TRF)"=w244:T17)
                      n182 = Unbundle(w301) -> ("compliance (A)"=w339:dbl, "compliance (V)"=w338:dbl)
                      n183 = local read "TRF Cluster"() -> (w292:T10)
                      n184 = Bundle("Start 3"=w306, "Stop 2"=w305, "Step 3"=w304, "sweep spacing (linear: 0)"=w343, "sweep mode"=w342, "compliance (V)"=w341, "compliance (A)"=w340) -> (w290:T18)  [unwired: 1 in]
                      n185 = local read "Sample Properties:"() -> (w241:T9)
                      n186 = local read "TRF Cluster"() -> (w303:T10)
                      n187 = Unbundle By Name(w303) -> ("Integration Time 3"=w288:u32)
                      n188 = Unbundle By Name(w292) -> ("Loop Step"=w295:dbl, "First Step"=w294:dbl)
                      n189 = local read "Saved Folder:"() -> (w260:path)
                      n190 = local write "Status Indicator"(TRUE) -> ()
                      n191 = Multiply(x=w295, y=w297) -> (x*y=w298:dbl)
                      n192 = Unbundle By Name(w241) -> ("Comments"=w243:string)
                      n193 = Add(x=w294, y=w298) -> (x+y=w293:dbl)
                      n194 = Bundle("compliance (A)"=w339, "compliance (V)"=w338, "Start 4"=w309, "Total Points 2"=w308, w293) -> (w289:T19)  [unwired: 1 in]
                      n195 = local read "Saved Folder:"() -> (w266:path)
                      n196 = Bundle By Name(cluster=w292, "Step 4"=w293) -> (w296:T10)
                      n197 = Build Path(base path=w260, name or relative path="TRF_SMU4") -> (appended path=w316:path)
                      n198 = Concatenate Strings(w243, "Gated SMU4" ("string")) -> (w240:string)
                      n199 = local write "TRF Cluster"(w296) -> ()
                      n200 = Build Path(base path=w260, name or relative path="LKG") -> (appended path=w256:path)
                      n201 = Bundle By Name(cluster=w241, "Comments"=w240) -> (w239:T9)
                      n202 = Unbundle(w239) -> ("Index (#)"=w334:string, "Index (ABC)"=w333:string, "Length"=w320:string, "Width"=w322:string, "T (K)"=w299:dbl)  [unwired: 8 out]
                      n203 = Decimal String To Number(string=w320) -> (number=w329:i32)  [unwired: 2 in, 1 out]
                      n204 = Concatenate Strings(w334, w333) -> (w251:string)
                      n205 = Equal?(x=w322, y=w323) -> (x = y?=w324:bool)
                      n206 = Number To Decimal String(number=w329) -> (decimal integer string=w325:string)  [unwired: 1 in]
                      n207 = Equal?(x=w320, y=w326) -> (x = y?=w327:bool)
                      n208 = Build Path(base path=w266, name or relative path="TRF") -> (appended path=w264:path)
                      n209 = Select(t=w326, s=w327, f=w325) -> (s? t:f=w250:string)
                      n210 = call <vilib>:"Check if File or Folder Exists.vi"("path"=w264) -> ("file or folder exists?"=w262:bool, "dup path"=w263:path)  [unwired: 8 in, 1 out]
                      n211 = local read "Graph Cluster"() -> (w282:T7)
                      n212 = property on="Status Indicator" class="Bool (strict)"("BoolText.Text"="Measuring\nTransfer (SMU4)") -> ()  [unwired: 2 in, 2 out]
                      n213 = case shown="False" w262 {
                        tunnel: w263 -> [w362 w363]
                        tunnel: [w361 w363] -> _
                        frame False {
                          n214 = Create Folder(path (use dialog)=w362) -> (created path=w361:path)  [unwired: 2 in, 2 out]
                        }
                        frame True {
                        }
                      }
                      n215 = Decimal String To Number(string=w322) -> (number=w328:i32)  [unwired: 2 in, 1 out]
                      n216 = Number To Decimal String(number=w328) -> (decimal integer string=w321:string)  [unwired: 1 in]
                      n217 = Select(t=w323, s=w324, f=w321) -> (s? t:f=w249:string)
                      n218 = Number To Decimal String(number=w299) -> (decimal integer string=w248:string)  [unwired: 1 in]
                      n219 = call "Build Text3"("T"=w248, "Index"=w251, "Length"=w250, "Width"=w249) -> ("Result"=w252:string)  [unwired: 10 in, 1 out]
                      n220 = call <vilib>:"Check if File or Folder Exists.vi"("path"=w316) -> ("file or folder exists?"=w318:bool, "dup path"=w317:path)  [unwired: 8 in, 1 out]
                      n221 = call <vilib>:"Check if File or Folder Exists.vi"("path"=w256) -> ("file or folder exists?"=w257:bool, "dup path"=w258:path)  [unwired: 8 in, 1 out]
                      n222 = call "Build Text"("T"=w248, "Index"=w251, "Length"=w250, "Width"=w249) -> ("Result"=w337:string)  [unwired: 10 in, 1 out]
                      n223 = case shown="False" w318 {
                        tunnel: w317 -> [w365 w366]
                        tunnel: [w364 w366] -> w315
                        frame False {
                          n224 = Create Folder(path (use dialog)=w365) -> (created path=w364:path)  [unwired: 2 in, 2 out]
                        }
                        frame True {
                        }
                      }
                      n225 = Build Path(base path=w315, name or relative path=w337) -> (appended path=w331:path)
                      n226 = case shown="False" w257 {
                        tunnel: w258 -> [w359 w360]
                        tunnel: [w358 w360] -> w247
                        frame False {
                          n227 = Create Folder(path (use dialog)=w359) -> (created path=w358:path)  [unwired: 2 in, 2 out]
                        }
                        frame True {
                        }
                      }
                      n228 = Build Path(base path=w247, name or relative path=w252) -> (appended path=w255:path)
                      n229 = call <vilib>:"Check if File or Folder Exists.vi"("path"=w331) -> ("file or folder exists?"=w332:bool, "dup path"=w330:path)  [unwired: 8 in, 1 out]
                      n230 = call <vilib>:"Check if File or Folder Exists.vi"("path"=w255) -> ("file or folder exists?"=w254:bool, "dup path"=w253:path)  [unwired: 8 in, 1 out]
                      n231 = case shown="True" w254 {
                        tunnel: w253 -> [w344 w346]
                        tunnel: [w344 w345] -> w246
                        frame False {
                        }
                        frame True {
                          n232 = while {
                            tunnel: w346 -> [w348]
                            tunnel: [w347] -> w345
                            i -> [w350]
                            stop <- w351 stop-if-true
                            n233 = Path To String(path=w348) -> (string=w357:string)
                            n234 = Increment(x=w350) -> (x+1=w349:i32)
                            n235 = Number To Decimal String(number=w349) -> (decimal integer string=w355:string)  [unwired: 1 in]
                            n236 = Concatenate Strings(w357, "_", w355) -> (w354:string)
                            n237 = String To Path(string=w354) -> (path=w353:path)
                            n238 = call <vilib>:"Check if File or Folder Exists.vi"("path"=w353) -> ("file or folder exists?"=w352:bool, "dup path"=w347:path)  [unwired: 8 in, 1 out]
                            n239 = Not(x=w352) -> (.not. x?=w351:bool)
                          }
                        }
                      }
                      n240 = case shown="True" w332 {
                        tunnel: w330 -> [w367 w369]
                        tunnel: [w367 w368] -> w287
                        frame False {
                        }
                        frame True {
                          n241 = while {
                            tunnel: w369 -> [w371]
                            tunnel: [w370] -> w368
                            i -> [w373]
                            stop <- w374 stop-if-true
                            n242 = Path To String(path=w371) -> (string=w380:string)
                            n243 = Increment(x=w373) -> (x+1=w372:i32)
                            n244 = Number To Decimal String(number=w372) -> (decimal integer string=w378:string)  [unwired: 1 in]
                            n245 = Concatenate Strings(w380, "_", w378) -> (w377:string)
                            n246 = String To Path(string=w377) -> (path=w376:path)
                            n247 = call <vilib>:"Check if File or Folder Exists.vi"("path"=w376) -> ("file or folder exists?"=w375:bool, "dup path"=w370:path)  [unwired: 8 in, 1 out]
                            n248 = Not(x=w375) -> (.not. x?=w374:bool)
                          }
                        }
                      }
                      n249 = call "transfer char run_subvi_SMU4_13_02_12_JWW.vi"("VISA session"=w291, "Y2 axis settings"=w244, "LKG Path"=w246, "Var1 sweep settings"=w290, "Var2 step settings"=w289, "integration time"=w288, "Input Path"=w287, "Dielectric Constant"=w238, "Sample Properties:"=w239) -> ("Check Cluster"=w284:T20, "Output"=w285:T21, "Graph Cluster"=w283:T22, "error?"=w286:errorcluster)  [unwired: 3 in]
                      n250 = local write "error out"(w286) -> ()
                      n251 = Unbundle By Name(w283) -> ("Linear Sqrt"=w281:cluster{dbl[], "trace":dbl[]}[], "Linear Log"=w280:cluster{dbl[], "trace":dbl[]}[], "Linear Raw"=w269:cluster{dbl[], dbl[]}[], "Saturation Sqrt"=w272:cluster{dbl[], "trace":dbl[]}[], "Saturation Log"=w271:cluster{dbl[], "trace":dbl[]}[], "Saturation Raw"=w268:cluster{dbl[], "trace":dbl[]}[], "Gate Current"=w261:cluster{dbl[], "trace":dbl[]}[])
                      n252 = Index Array(array=w281, index=w279) -> (element=w278:cluster{dbl[], "trace":dbl[]})
                      n253 = Index Array(array=w280, index=w279) -> (element=w277:cluster{dbl[], "trace":dbl[]})
                      n254 = Index Array(array=w272, index=w273) -> (element=w274:cluster{dbl[], "trace":dbl[]})
                      n255 = Index Array(array=w271, index=w273) -> (element=w275:cluster{dbl[], "trace":dbl[]})
                      n256 = Build Array(w278, w277) -> (w276:cluster{dbl[], "trace":dbl[]}[])
                      n257 = Build Array(w274, w275) -> (w270:cluster{dbl[], "trace":dbl[]}[])
                      n258 = Bundle By Name(cluster=w282, "Linear Transfer"=w276, "Linear Raw"=w269, "Saturation Transfer"=w270, "Saturation Raw"=w268, "TRF Gate Current"=w261) -> (w267:T7)
                      n259 = local write "Graph Cluster"(w267) -> ()
                      n260 = local write "Vt Cluster"(w284) -> ()
                      n261 = local write "Char Cluster"(w285) -> ()
                      n262 = property on="Saturation Transfer" class="XYGraph (strict)"("Active Plot"=0, "Plot.YScaleIdx"=0, "Active Plot"=1, "Plot.YScaleIdx"=0) -> ()  [unwired: 2 in, 2 out]
                      n263 = local write "LKG Path"(w246) -> ()
                      n264 = local write "TRF Path"(w287) -> ()
                    }
                  }
                }
              }
            }
          }
        }
        frame #3 {
          n265 = local write "Status Indicator"(FALSE) -> ()
        }
        frame #4 {
          # "This frame creates the countdown timer for the wait inbetween the\nTransfer and Transport (if both selected)."
          n266 = disable-structure shown="Disabled" {
            frame Disabled {
              n267 = node-c288(1) -> (w395:T12)  [unwired: 1 in]
              n268 = timed-loop {
                timing: w395 -> [_]
                timing-out: [_] -> w394
                i -> [w406]
                stop <- w407 stop-if-true
                n269 = node-c288() -> ()  [unwired: 1 in, 1 out]
                n270 = local read "Wait Cluster"() -> (w399:T5)
                n271 = Unbundle By Name(w399) -> ("Wait Time (s)"=w397:dbl)
                n272 = Multiply(x=w406, y=0.001) -> (x*y=w404:dbl)
                n273 = local read "TRF Cluster"() -> (w400:T10)
                n274 = local read "TSP Cluster"() -> (w401:T11)
                n275 = Unbundle By Name(w401) -> ("Transport"=w402:bool)
                n276 = Unbundle By Name(w400) -> ("Transfer 2"=w403:bool)
                n277 = And(x=w403, y=w402) -> (x .and. y?=w411:bool)
                n278 = Select(t="Waiting...", s=w411, f="Ready") -> (s? t:f=w413:string)
                n279 = property on="Status Indicator" class="Bool (strict)"("BoolText.Text"=w413) -> ()  [unwired: 2 in, 2 out]
                n280 = Select(t=w397, s=w411, f=0) -> (s? t:f=w409:dbl)
                n281 = Subtract(x=w409, y=w404) -> (x-y=w398:dbl)
                n282 = Less Or Equal?(x=w398, y=0) -> (x <= y?=w407:bool)
                n283 = Bundle("Wait Time (s)"=w397, w398) -> (w396:cluster{"Wait Time (s)":dbl, dbl})  [unwired: 1 in]
                n284 = local write "Wait Cluster"(w396) -> ()
                n285 = node-c288() -> ()  [unwired: 1 in, 1 out]
              }
              n286 = node-c288(w394) -> ()  [unwired: 1 out]
            }
            frame Enabled {
            }
          }
          n287 = local read "Light Bathe Cluster"() -> (w382:T2)
          n288 = Unbundle By Name(w382) -> ("TRF to TSP:"=w385:bool, "TRF to TSP Duration"=w384:dbl)
          n289 = local read "VISA resource name"() -> (w383:refnum<visa-resource-name>)
          n290 = case shown="True" w385 {
            tunnel: w384 -> [_ w387]
            tunnel: w383 -> [_ w386]
            frame False {
            }
            frame True {
              n291 = flat-sequence {
                tunnel: w386 -> [w388]
                tunnel: w387 -> [w390]
                tunnel: w386 -> [w391]
                frame #0 {
                  w389 = u32 1 items=["positive pulse  ", "negative pulse  ", "level high  ", "level low  "] ("trigger signal")
                  n292 = call "HP415xA Op-Trigger Output.vi"("trigger signal"=w389, "VISA session"=w388) -> ()  [unwired: 2 in, 1 out]
                }
                frame #1 {
                  n293 = call "Time Delay2"("Delay Time (s)"=w390) -> ()  [unwired: 10 in, 1 out]
                }
                frame #2 {
                  w392 = u32 0 items=["positive pulse  ", "negative pulse  ", "level high  ", "level low  "] ("trigger signal")
                  n294 = call "HP415xA Op-Trigger Output.vi"("trigger signal"=w392, "VISA session"=w391) -> ()  [unwired: 2 in, 1 out]
                }
              }
            }
          }
        }
        frame #5 {
          n295 = local read "TSP Cluster"() -> (w422:T11)
          n296 = Unbundle By Name(w422) -> ("Transport"=w421:bool)
          n297 = case shown="True" w421 {
            frame False {
            }
            frame True {
              n298 = stacked-sequence {
                frame #0 {
                  w455 = "XXX"
                  w459 = "XXX"
                  # "TSP w/o SMU4"
                  # "This frame takes the measurement settings and sends them to the Transport subVI for execution (if the \"Transport\" checkbox is selected on the front panel).\n\nThe data is saved to the folder specified by the user on the front panel with the file name generated by the sample properties.  If the file name already exists, the data is appended to the end of the file.\n\nThe Indicator LED on the front panel should display \"Measuring Transport\"."
                  n299 = local read "Compliance Cluster"() -> (w434:T6)
                  n300 = local read "TSP Cluster"() -> (w446:T11)
                  n301 = local read "Gate Current Cluster"() -> (w424:T3)
                  n302 = Unbundle By Name(w434) -> ("Var1 sweep settings 2"=w433:T15, "Var2 step settings 2"=w432:T16)
                  n303 = local read "TSP Cluster"() -> (w439:T11)
                  n304 = local read "VISA resource name"() -> (w436:refnum<visa-resource-name>)
                  n305 = local read "TSP Cluster"() -> (w437:T11)
                  n306 = Unbundle By Name(w437) -> ("Start"=w442:dbl, "Total Points"=w441:u16, "Step"=w440:dbl)
                  n307 = Unbundle By Name(w446) -> ("Start 2"=w445:dbl, "Stop 3"=w444:dbl, "Step 2"=w443:dbl)
                  n308 = Unbundle By Name(w439) -> ("Integration Time"=w438:u32)
                  n309 = Unbundle By Name(w424) -> ("Gate Current (TSP)"=w423:T17)
                  n310 = Unbundle(w433) -> ("sweep spacing (linear: 0)"=w482:u16, "sweep mode"=w481:bool, "compliance (V)"=w480:dbl, "compliance (A)"=w479:dbl)
                  n311 = Bundle("Start 2"=w445, "Stop 3"=w444, "Step 2"=w443, "sweep spacing (linear: 0)"=w482, "sweep mode"=w481, "compliance (V)"=w480, "compliance (A)"=w479) -> (w478:T23)  [unwired: 1 in]
                  n312 = Unbundle(w432) -> ("compliance (A)"=w477:dbl, "compliance (V)"=w476:dbl)
                  n313 = local read "Saved Folder:"() -> (w435:path)
                  n314 = Bundle("compliance (A)"=w477, "compliance (V)"=w476, "Start"=w442, "Total Points"=w441, "Step"=w440) -> (w475:T24)  [unwired: 1 in]
                  n315 = local read "Sample Properties:"() -> (w471:T9)
                  n316 = local write "Status Indicator"(TRUE) -> ()
                  n317 = Build Path(base path=w435, name or relative path="TSP") -> (appended path=w448:path)
                  n318 = Unbundle(w471) -> ("Index (#)"=w470:string, "Index (ABC)"=w469:string, "Length"=w460:string, "Width"=w456:string, "T (K)"=w430:dbl)  [unwired: 8 out]
                  n319 = Equal?(x=w459, y=w460) -> (x = y?=w461:bool)
                  n320 = property on="Status Indicator" class="Bool (strict)"("BoolText.Text"="Measuring\nTransport") -> ()  [unwired: 2 in, 2 out]
                  n321 = Concatenate Strings(w470, w469) -> (w468:string)
                  n322 = Equal?(x=w455, y=w456) -> (x = y?=w464:bool)
                  n323 = local read "Graph Cluster"() -> (w428:T7)
                  n324 = Decimal String To Number(string=w460) -> (number=w463:i32)  [unwired: 2 in, 1 out]
                  n325 = Decimal String To Number(string=w456) -> (number=w462:i32)  [unwired: 2 in, 1 out]
                  n326 = call <vilib>:"Check if File or Folder Exists.vi"("path"=w448) -> ("file or folder exists?"=w450:bool, "dup path"=w449:path)  [unwired: 8 in, 1 out]
                  n327 = case shown="False" w450 {
                    tunnel: w449 -> [w484 w485]
                    tunnel: [w483 w485] -> w447
                    frame False {
                      n328 = Create Folder(path (use dialog)=w484) -> (created path=w483:path)  [unwired: 2 in, 2 out]
                    }
                    frame True {
                    }
                  }
                  n329 = Number To Decimal String(number=w463) -> (decimal integer string=w458:string)  [unwired: 1 in]
                  n330 = Select(t=w459, s=w461, f=w458) -> (s? t:f=w457:string)
                  n331 = Number To Decimal String(number=w462) -> (decimal integer string=w454:string)  [unwired: 1 in]
                  n332 = Select(t=w455, s=w464, f=w454) -> (s? t:f=w453:string)
                  n333 = call "Build Text2"("T"=w430, "Index"=w468, "Length"=w457, "Width"=w453) -> ("Result"=w452:string)  [unwired: 10 in, 1 out]
                  n334 = Build Path(base path=w447, name or relative path=w452) -> (appended path=w465:path)
                  n335 = call <vilib>:"Check if File or Folder Exists.vi"("path"=w465) -> ("file or folder exists?"=w467:bool, "dup path"=w466:path)  [unwired: 8 in, 1 out]
                  n336 = case shown="True" w467 {
                    tunnel: w466 -> [w486 w488]
                    tunnel: [w486 w487] -> w431
                    frame False {
                    }
                    frame True {
                      n337 = while {
                        tunnel: w488 -> [w490]
                        tunnel: [w489] -> w487
                        i -> [w492]
                        stop <- w493 stop-if-true
                        n338 = Path To String(path=w490) -> (string=w499:string)
                        n339 = Increment(x=w492) -> (x+1=w491:i32)
                        n340 = Number To Decimal String(number=w491) -> (decimal integer string=w497:string)  [unwired: 1 in]
                        n341 = Concatenate Strings(w499, "_", w497) -> (w496:string)
                        n342 = String To Path(string=w496) -> (path=w495:path)
                        n343 = call <vilib>:"Check if File or Folder Exists.vi"("path"=w495) -> ("file or folder exists?"=w494:bool, "dup path"=w489:path)  [unwired: 8 in, 1 out]
                        n344 = Not(x=w494) -> (.not. x?=w493:bool)
                      }
                    }
                  }
                  n345 = call "transport char run_subvi_2013_09_11_JWa.vi"("VISA session"=w436, "Y2 axis settings"=w423, "Var1 sweep settings"=w478, "Var2 step settings"=w475, "integration time"=w438, "Path"=w431, "Sample Properties:"=w471) -> ("Graph Cluster"=w429:T25, "error?"=w474:errorcluster)  [unwired: 6 in, 1 out]
                  n346 = local write "error out"(w474) -> ()
                  n347 = Unbundle By Name(w429) -> ("Transport"=w426:cluster{dbl[], dbl[]}[], "Gate Current"=w425:cluster{dbl[], dbl[]}[])
                  n348 = local write "TSP Path"(w431) -> ()
                  n349 = Bundle By Name(cluster=w428, "Transport"=w426, "TSP Gate Current"=w425) -> (w427:T7)
                  n350 = local write "Graph Cluster"(w427) -> ()
                }
                frame #1 {
                  n351 = local read "Gated SMU4 is..."() -> (w500:bool)
                  n352 = case shown="True" w500 {
                    frame False {
                    }
                    frame True {
                      n353 = local read "Light Bathe Cluster"() -> (w504:T2)
                      n354 = local read "VISA resource name"() -> (w501:refnum<visa-resource-name>)
                      n355 = Unbundle By Name(w504) -> ("TG to BG (TSP):"=w503:bool, "TG to BG Durration 3"=w502:dbl)
                      n356 = case shown="True" w503 {
                        tunnel: w502 -> [_ w506]
                        tunnel: w501 -> [_ w505]
                        frame False {
                        }
                        frame True {
                          n357 = flat-sequence {
                            tunnel: w505 -> [w507]
                            tunnel: w506 -> [w509]
                            tunnel: w505 -> [w510]
                            frame #0 {
                              w508 = u32 1 items=["positive pulse  ", "negative pulse  ", "level high  ", "level low  "] ("trigger signal")
                              n358 = call "HP415xA Op-Trigger Output.vi"("trigger signal"=w508, "VISA session"=w507) -> ()  [unwired: 2 in, 1 out]
                            }
                            frame #1 {
                              n359 = call "Time Delay3"("Delay Time (s)"=w509) -> ()  [unwired: 10 in, 1 out]
                            }
                            frame #2 {
                              w511 = u32 0 items=["positive pulse  ", "negative pulse  ", "level high  ", "level low  "] ("trigger signal")
                              n360 = call "HP415xA Op-Trigger Output.vi"("trigger signal"=w511, "VISA session"=w510) -> ()  [unwired: 2 in, 1 out]
                            }
                          }
                        }
                      }
                    }
                  }
                }
                frame #2 {
                  # "TSP w/ SMU4"
                  n361 = local read "Gated SMU4 is..."() -> (w512:bool)
                  n362 = case shown="True" w512 {
                    frame False {
                    }
                    frame True {
                      w545 = "XXX"
                      w549 = "XXX"
                      # "This frame takes the measurement settings and sends them to the Transport subVI for execution (if the \"Transport\" checkbox is selected on the front panel).\n\nThe data is saved to the folder specified by the user on the front panel with the file name generated by the sample properties.  If the file name already exists, the data is appended to the end of the file.\n\nThe Indicator LED on the front panel should display \"Measuring Transport\"."
                      n363 = local read "Compliance Cluster"() -> (w524:T6)
                      n364 = local read "TSP Cluster"() -> (w536:T11)
                      n365 = local read "Gate Current Cluster"() -> (w514:T3)
                      n366 = Unbundle By Name(w524) -> ("Var1 sweep settings 2"=w523:T15, "Var2 step settings 2"=w522:T16)
                      n367 = local read "TSP Cluster"() -> (w529:T11)
                      n368 = local read "VISA resource name"() -> (w526:refnum<visa-resource-name>)
                      n369 = local read "TSP Cluster"() -> (w527:T11)
                      n370 = Unbundle By Name(w527) -> ("Start"=w532:dbl, "Total Points"=w531:u16, "Step"=w530:dbl)
                      n371 = Unbundle By Name(w536) -> ("Start 2"=w535:dbl, "Stop 3"=w534:dbl, "Step 2"=w533:dbl)
                      n372 = Unbundle By Name(w529) -> ("Integration Time"=w528:u32)
                      n373 = Unbundle By Name(w514) -> ("Gate Current (TSP)"=w513:T17)
                      n374 = Unbundle(w523) -> ("sweep spacing (linear: 0)"=w572:u16, "sweep mode"=w571:bool, "compliance (V)"=w570:dbl, "compliance (A)"=w569:dbl)
                      n375 = Bundle("Start 2"=w535, "Stop 3"=w534, "Step 2"=w533, "sweep spacing (linear: 0)"=w572, "sweep mode"=w571, "compliance (V)"=w570, "compliance (A)"=w569) -> (w568:T23)  [unwired: 1 in]
                      n376 = Unbundle(w522) -> ("compliance (A)"=w567:dbl, "compliance (V)"=w566:dbl)
                      n377 = local read "Saved Folder:"() -> (w525:path)
                      n378 = Bundle("compliance (A)"=w567, "compliance (V)"=w566, "Start"=w532, "Total Points"=w531, "Step"=w530) -> (w565:T24)  [unwired: 1 in]
                      n379 = local read "Sample Properties:"() -> (w561:T9)
                      n380 = local write "Status Indicator"(TRUE) -> ()
                      n381 = Build Path(base path=w525, name or relative path="TSP_SMU4") -> (appended path=w538:path)
                      n382 = Unbundle(w561) -> ("Index (#)"=w560:string, "Index (ABC)"=w559:string, "Length"=w550:string, "Width"=w546:string, "T (K)"=w520:dbl)  [unwired: 8 out]
                      n383 = Equal?(x=w549, y=w550) -> (x = y?=w551:bool)
                      n384 = property on="Status Indicator" class="Bool (strict)"("BoolText.Text"="     Measuring\nTransport SMU4") -> ()  [unwired: 2 in, 2 out]
                      n385 = Concatenate Strings(w560, w559) -> (w558:string)
                      n386 = Equal?(x=w545, y=w546) -> (x = y?=w554:bool)
                      n387 = local read "Graph Cluster"() -> (w518:T7)
                      n388 = Decimal String To Number(string=w550) -> (number=w553:i32)  [unwired: 2 in, 1 out]
                      n389 = Decimal String To Number(string=w546) -> (number=w552:i32)  [unwired: 2 in, 1 out]
                      n390 = call <vilib>:"Check if File or Folder Exists.vi"("path"=w538) -> ("file or folder exists?"=w540:bool, "dup path"=w539:path)  [unwired: 8 in, 1 out]
                      n391 = case shown="False" w540 {
                        tunnel: w539 -> [w574 w575]
                        tunnel: [w573 w575] -> w537
                        frame False {
                          n392 = Create Folder(path (use dialog)=w574) -> (created path=w573:path)  [unwired: 2 in, 2 out]
                        }
                        frame True {
                        }
                      }
                      n393 = Number To Decimal String(number=w553) -> (decimal integer string=w548:string)  [unwired: 1 in]
                      n394 = Select(t=w549, s=w551, f=w548) -> (s? t:f=w547:string)
                      n395 = Number To Decimal String(number=w552) -> (decimal integer string=w544:string)  [unwired: 1 in]
                      n396 = Select(t=w545, s=w554, f=w544) -> (s? t:f=w543:string)
                      n397 = call "Build Text6"("T"=w520, "Index"=w558, "Length"=w547, "Width"=w543) -> ("Result"=w542:string)  [unwired: 10 in, 1 out]
                      n398 = Build Path(base path=w537, name or relative path=w542) -> (appended path=w555:path)
                      n399 = call <vilib>:"Check if File or Folder Exists.vi"("path"=w555) -> ("file or folder exists?"=w557:bool, "dup path"=w556:path)  [unwired: 8 in, 1 out]
                      n400 = case shown="True" w557 {
                        tunnel: w556 -> [w576 w578]
                        tunnel: [w576 w577] -> w521
                        frame False {
                        }
                        frame True {
                          n401 = while {
                            tunnel: w578 -> [w580]
                            tunnel: [w579] -> w577
                            i -> [w582]
                            stop <- w583 stop-if-true
                            n402 = Path To String(path=w580) -> (string=w589:string)
                            n403 = Increment(x=w582) -> (x+1=w581:i32)
                            n404 = Number To Decimal String(number=w581) -> (decimal integer string=w587:string)  [unwired: 1 in]
                            n405 = Concatenate Strings(w589, "_", w587) -> (w586:string)
                            n406 = String To Path(string=w586) -> (path=w585:path)
                            n407 = call <vilib>:"Check if File or Folder Exists.vi"("path"=w585) -> ("file or folder exists?"=w584:bool, "dup path"=w579:path)  [unwired: 8 in, 1 out]
                            n408 = Not(x=w584) -> (.not. x?=w583:bool)
                          }
                        }
                      }
                      n409 = call "transport char run_subvi_2014_02_18_SMU4_JWa.vi"("VISA session"=w526, "Y2 axis settings"=w513, "Var1 sweep settings"=w568, "Var2 step settings"=w565, "integration time"=w528, "Path"=w521, "Sample Properties:"=w561) -> ("Graph Cluster"=w519:T25, "error?"=w564:errorcluster)  [unwired: 6 in, 1 out]
                      n410 = local write "error out"(w564) -> ()
                      n411 = Unbundle By Name(w519) -> ("Transport"=w516:cluster{dbl[], dbl[]}[], "Gate Current"=w515:cluster{dbl[], dbl[]}[])
                      n412 = local write "TSP Path"(w521) -> ()
                      n413 = Bundle By Name(cluster=w518, "Transport"=w516, "TSP Gate Current"=w515) -> (w517:T7)
                      n414 = local write "Graph Cluster"(w517) -> ()
                    }
                  }
                }
              }
            }
          }
        }
        frame #6 {
          n415 = local write "Status Indicator"(FALSE) -> ()
          n416 = property on="Status Indicator" class="Bool (strict)"("BoolText.Text"="Ready") -> ()  [unwired: 2 in, 2 out]
        }
        frame #7 {
          n417 = disable-structure shown="Disabled" {
            disable-tunnel: w593 -> [w595 _]
            disable-tunnel: w592 -> [w594 _]
            frame Disabled {
              n418 = node-c288(100) -> (w600:T12)  [unwired: 3 in]
              n419 = timed-loop {
                timing: w600 -> [_]
                timing-out: [_] -> w599
                tunnel: w595 -> [w611]
                tunnel: w594 -> [w610]
                tunnel: ["Stop \nCountdown"] -> _
                i -> [w616]
                stop <- w606 stop-if-true
                n420 = node-c288() -> ()  [unwired: 1 in, 1 out]
                n421 = local read "TRF Cluster"() -> (w605:T10)
                n422 = Unbundle By Name(w605) -> ("Loop Wait"=w603:dbl)
                n423 = Multiply(x=0.1, y=w616) -> (x*y=w614:dbl)
                n424 = Equal?(x=w610, y=w611) -> (x = y?=w612:bool)
                n425 = Select(t=0, s=w612, f=w603) -> (s? t:f=w608:dbl)
                n426 = Subtract(x=w608, y=w614) -> (x-y=w602:dbl)
                n427 = Less Or Equal To 0?(x=w602) -> (x <= 0?=w607:bool)
                n428 = Or(x=w607, y="Stop \nCountdown") -> (x .or. y?=w606:bool)
                n429 = Bundle("Loop Wait"=w603, w602) -> (w604:cluster{"Loop Wait":dbl, dbl})  [unwired: 1 in]
                n430 = property on="Status Indicator" class="Bool (strict)"("BoolText.Text"="Waiting...") -> ()  [unwired: 2 in, 2 out]
                n431 = local write "Wait Cluster"(w604) -> ()
                n432 = node-c288() -> ()  [unwired: 1 in, 1 out]
              }
              n433 = node-c288(w599) -> (w596:errorcluster)
              n434 = property on="Status Indicator" class="Bool (strict)"(error in=w596, "BoolText.Text"="Ready") -> ()  [unwired: 1 in, 2 out]
            }
            frame Enabled {
            }
          }
        }
      }
      n435 = local write "VISA resource name out"(w9) -> ()
    }
  }
